vi "Match idot to shot utility.vi"(6 "Shots file":path=path "Z:/ShotHistory2014.txt", 7 "Log file folder":path=path "C:/Data", 8 "error in (no error)":errorcluster, 10 "Idot match record":T1, 11 "Root Data Folder":path=path "C:/Data") -> (0 "error out":errorcluster, 2 "Formated shot data":string, 3 "File output":path)   [LabVIEW 2015]
uses:
  Mag Lab Measure/Mag Lab Measure Controller/Cap Bank Server/Idot match record.ctl
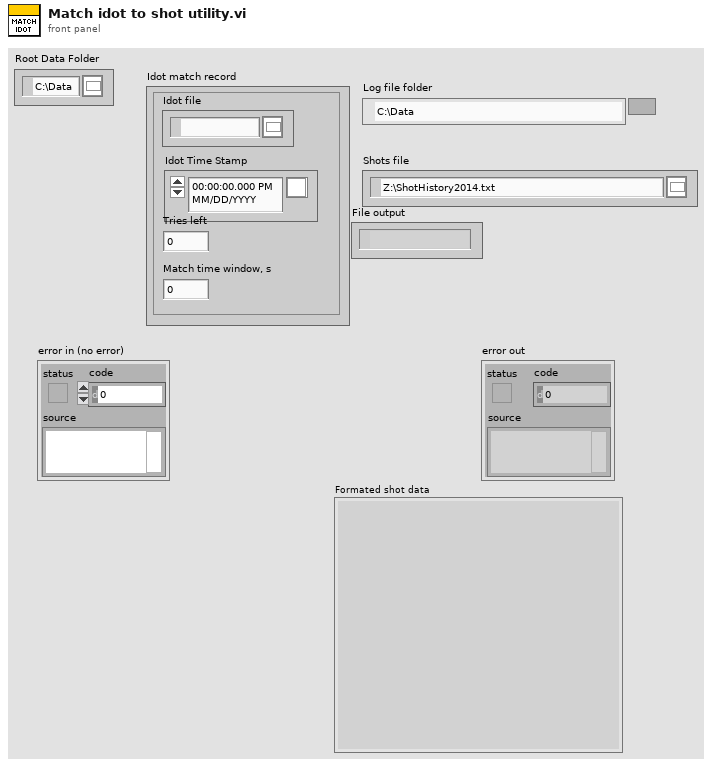
[diagram p1: front panel]
types:
  T1 = typedef "Idot match record.ctl" = cluster{"Idot file":path, "Idot Time Stamp":timestamp, "Tries left":i32, "Match time window, s":dbl}
  T2 = typedef "Shot data.ctl" = cluster{"Shot number":i32, "Time":timestamp, "Magnet ID":string, "User":string, "Cell number":i32, "Requested field":dbl, "Field direction":string, "Number of bank frames":i32, "Crowbar resistance, mOhm":dbl, "Magnet resistance, mOhm":dbl, "Charger voltage, kV":dbl, "Frame voltage, kV":dbl}
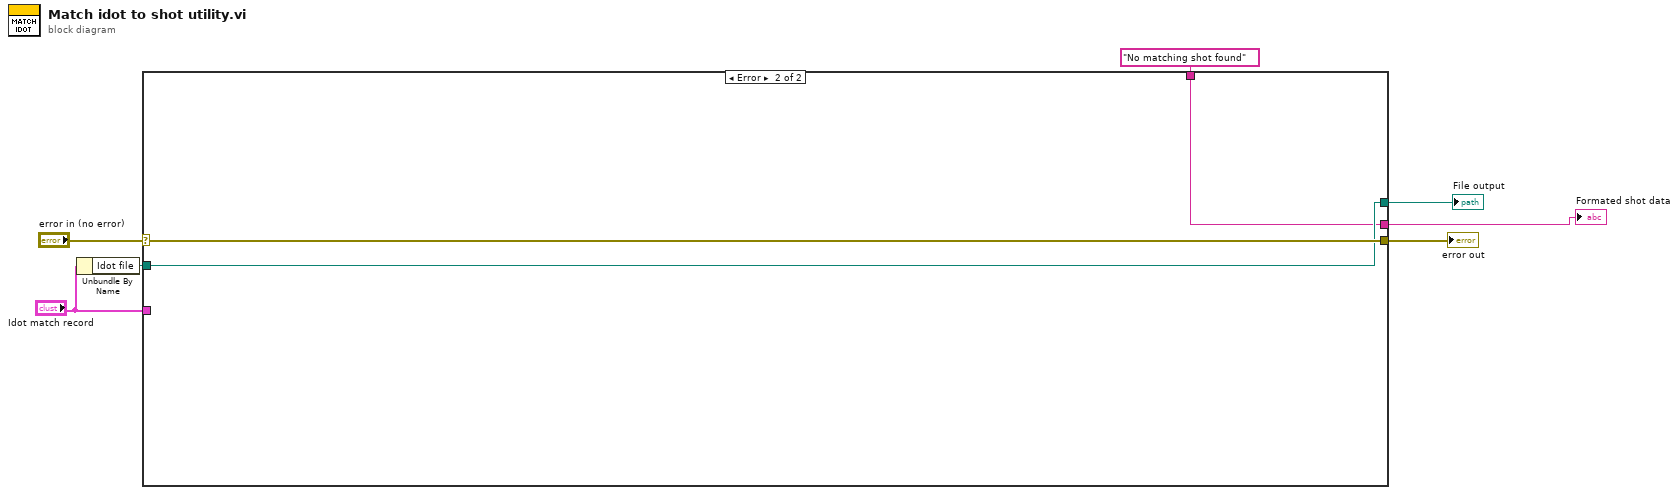
[diagram p0: block diagram]
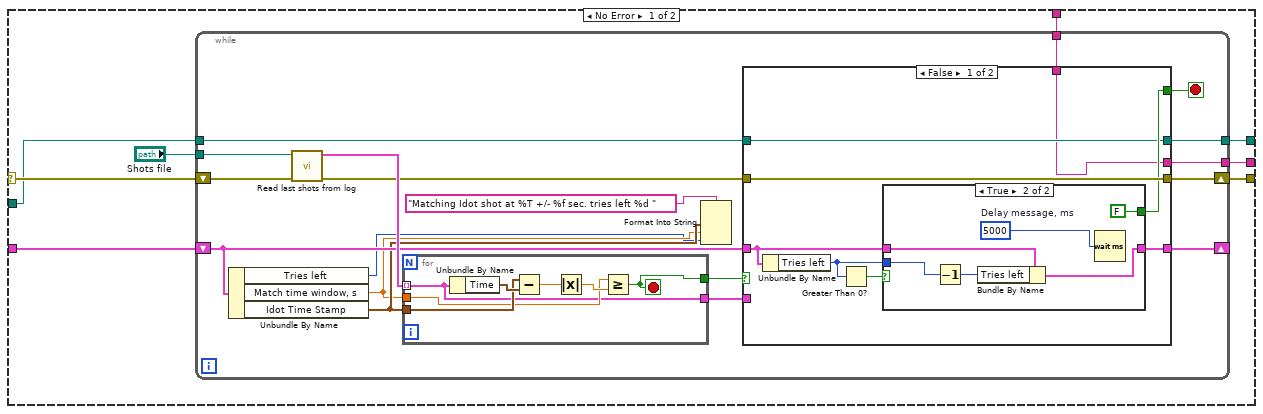
[diagram p2: hidden frame]
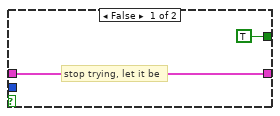
[diagram p3: hidden frame]
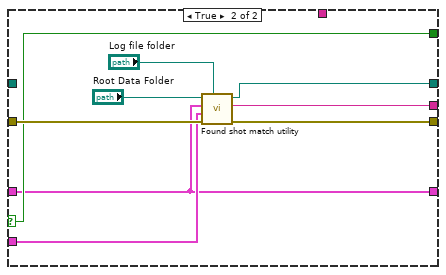
[diagram p4: hidden frame]
diagram:
  n1 = Unbundle By Name("Idot match record") -> ("Idot file"=w3:path)
  n2 = case shown="Error" "error in (no error)" {
    selector: "error in (no error)" -> [w15 w68]
    tunnel: [w14 w68] -> w6
    tunnel: [w12 w67] -> w5
    tunnel: "Idot match record" -> [w11 _]
    tunnel: w3 -> [w10 w67]
    tunnel: [w9 w66] -> w2
    tunnel: "No matching shot found" ("Formated shot data") -> [w8 w66]
    frame No Error {
      n3 = while {
        tunnel: "Shots file" -> [w23]
        shift-right: [w30] -> w14
        shift-left: w15 -> [w32]
        shift-right: [w21] -> _
        shift-left: w11 -> [w28]
        tunnel: [w19] -> w12
        tunnel: w10 -> [w18]
        tunnel: [w17] -> w9
        tunnel: w8 -> [w16]
        stop <- w22 stop-if-true
        n4 = Unbundle By Name(w28) -> ("Tries left"=w24:i32, "Match time window, s"=w25:dbl, "Idot Time Stamp"=w27:timestamp)
        n5 = call "Read last shots from log.vi"("Error In"=w32, "Shots file"=w23) -> ("Error Out"=w20:errorcluster, "Last shots"=w33:T2[])  [unwired: 6 in, 2 out]
        n6 = for {
          tunnel: w33 -> [w59] mode=indexing
          tunnel: w27 -> [w64]
          tunnel: w25 -> [w61]
          tunnel: [w60] -> w31
          tunnel: [w59] -> w29
          stop <- w60 stop-if-true
          n7 = Unbundle By Name(w59) -> ("Time"=w65:timestamp)
          n8 = Subtract(x=w64, y=w65) -> (x-y=w63:dbl)
          n9 = Absolute Value(x=w63) -> (abs(x)=w62:dbl)
          n10 = Greater Or Equal?(x=w61, y=w62) -> (x >= y?=w60:bool)
        }
        n11 = Format Into String(format string="Matching Idot shot at %T +/- %f sec. tries left %d " ("Status"), w27, w25, w24) -> ()  [unwired: 2 in, 2 out]
        n12 = case shown="False" w31 {
          selector: w31 -> [_ w55]
          tunnel: w20 -> [w41 w58]
          tunnel: [w41 w57] -> w30
          tunnel: w29 -> [_ w56]
          tunnel: w28 -> [w40 w54]
          tunnel: [w37 w55] -> w22
          tunnel: [w36 w54] -> w21
          tunnel: [w35 w51] -> w19
          tunnel: w18 -> [w35 _]
          tunnel: [w34 w50] -> w17
          tunnel: w16 -> [w34 _]
          frame False {
            n13 = Unbundle By Name(w40) -> ("Tries left"=w38:i32)
            n14 = Greater Than 0?(x=w38) -> (x > 0?=w39:bool)
            n15 = case shown="True" w39 {
              tunnel: w40 -> [w42 w48]
              tunnel: w38 -> [_ w46]
              tunnel: [TRUE FALSE] -> w37
              tunnel: [w42 w44] -> w36
              frame False {
                # "stop trying, let it be"
              }
              frame True {
                w49 = u32 5000  # Delay message, ms
                n16 = Decrement(x=w46) -> (x-1=w47:i32)
                n17 = Bundle By Name(cluster=w48, "Tries left"=w47) -> (w44:T1)
                n18 = Wait (ms)(milliseconds to wait=w49) -> ()  [unwired: 1 out]
              }
            }
          }
          frame True {
            n19 = call "Found shot match utility.vi"("Log file folder"="Log file folder", "error in (no error)"=w58, "Shot data"=w56, "Idot match record"=w54, "Root Data Folder"="Root Data Folder") -> ("error out"=w57:errorcluster, "Formated shot data"=w50:string, "File output"=w51:path)  [unwired: 4 in]
          }
        }
      }
    }
    frame Error {
    }
  }
  "error out" <- w6
  "File output" <- w5
  "Formated shot data" <- w2
